vi "Write Is Static.vi"(8 "error in (no error)":errorcluster, 10 "Is Static":bool, 11 "Collider in":refnum<class "Collider.lvclass">) -> (0 "error out":errorcluster, 3 "Collider out":refnum<class "Collider.lvclass">)   [LabVIEW 2022 SP3, in "Collider.lvclass"]
uses:
  Collider.lvclass
  Collider.lvclass/Collider.ctl
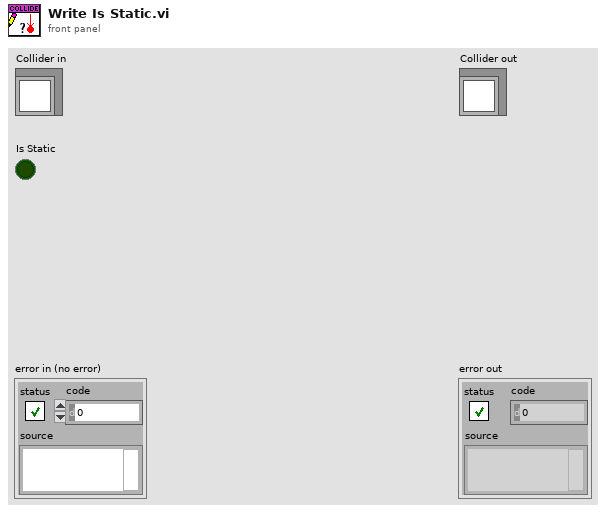
[diagram p1: front panel]
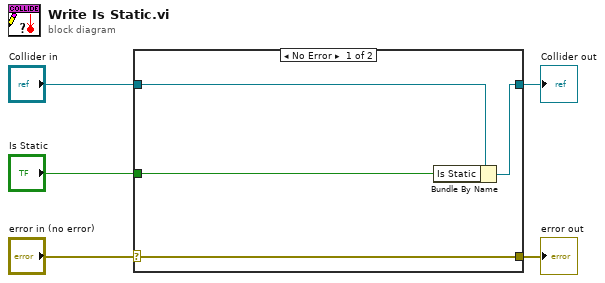
[diagram p0: block diagram]
diagram:
  n1 = case shown="No Error" "error in (no error)" {
    selector: "error in (no error)" -> [w9 w10]
    tunnel: [w9 w10] -> w4
    tunnel: [w7 w11] -> w2
    tunnel: "Collider in" -> [w8 w11]
    tunnel: "Is Static" -> [w6 _]
    frame No Error {
      n2 = Bundle By Name(cluster=w8, "Is Static"=w6) -> (w7:refnum<class "Collider.lvclass">)
    }
    frame Error {
    }
  }
  "error out" <- w4
  "Collider out" <- w2
